vi "get_num_elements.vi"(9 "item offset":i32, 11 "TypeDescriptor":refnum<class "TD.lvclass">) -> (2 "num_element":i32, 3 "TypeDescriptor out":refnum<class "TD.lvclass">)   [LabVIEW 2020, in "variant.lvlib" / "type.lvlib" / "TD.lvclass"]
uses:
  TD.lvclass
  C:/projects/OpenG-Variant-Data-Library/source/library/Bytes/Bytes.lvclass
  Bytes/Bytes.lvclass/Bytes.ctl
  b3898c1b-5169-4cb1-894b-457c92b4a1c3.vi
  b3898c1b-5169-4cb1-894b-457c92b4a1c3.vi/81433c74-ee36-47cf-a886-10c868675b30.vi
  b3898c1b-5169-4cb1-894b-457c92b4a1c3.vi/d8d9ff34-2c15-4edb-a5ad-7260f11560db.vi
  Bytes/read.vi
  Bytes/to_data.vi
  Bytes/from_byte_array.vi
  Bytes/Bytes.lvclass
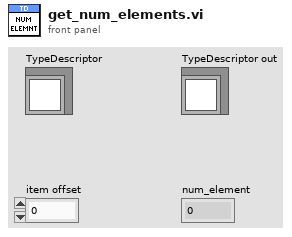
[diagram p1: front panel]
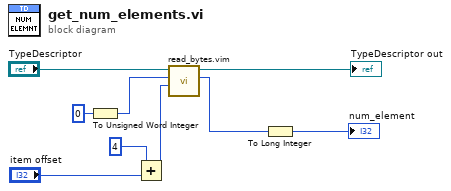
[diagram p0: block diagram]
diagram:
  n1 = To Unsigned Word Integer(number=i16 0 ("data type")) -> (unsigned 16bit integer=w7:u16)
  n2 = Add(x=4 ("byte offset"), y="item offset") -> (x+y=w1:i32)
  n3 = call "read_bytes.vim"("byte offset"=w1, "data type"=w7, "Bytes in"="TypeDescriptor") -> ("value"=w6:u16, "Bytes out"=→"TypeDescriptor out":refnum<class "TD.lvclass">)  [unwired: 7 in]
  n4 = To Long Integer(number=w6) -> (32bit integer=→"num_element":i32)
